vi "SET Project Editor.vi"() -> ()   [LabVIEW 2013]
uses:
  Lib/Splash/SET_Splash.lvlib
panel:
  out "Status":string=" "
  # "SET Localization Project Editor"
  # "Edit-time language switching toolkit for NI LabVIEW\"! 2013"
  # "Version 0.4.0"
  # "Copyright © 2014, Ryan Porter. All rights reserved."
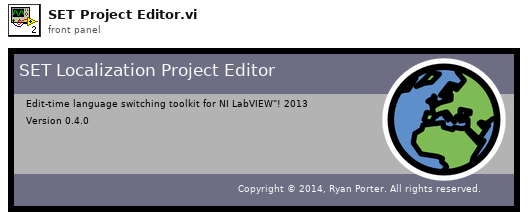
[diagram p1: front panel]
types:
  T1 = enum32{"Invalid", "Standard", "Closed", "Hidden", "Minimized", "Maximized"}
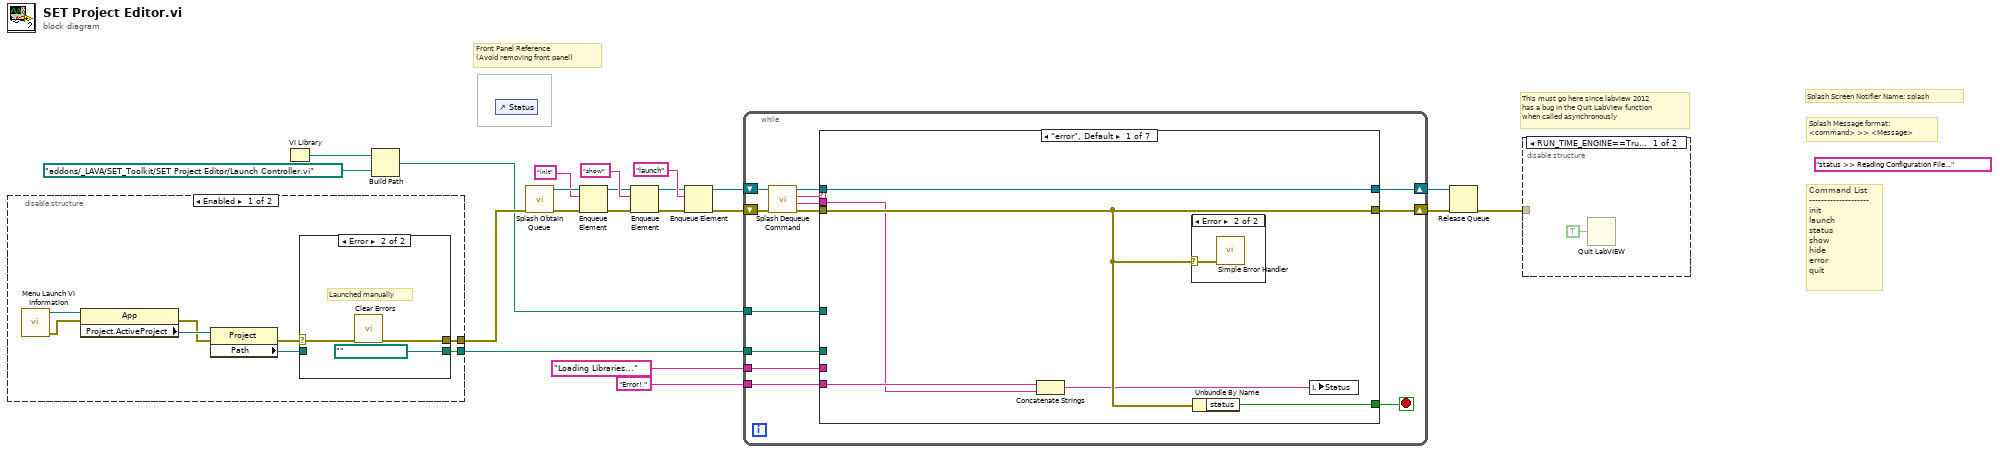
[diagram p0: block diagram]
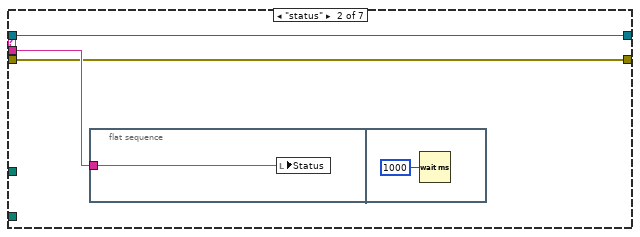
[diagram p3: hidden frame]
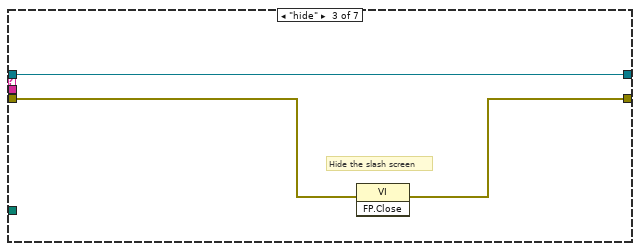
[diagram p4: hidden frame]
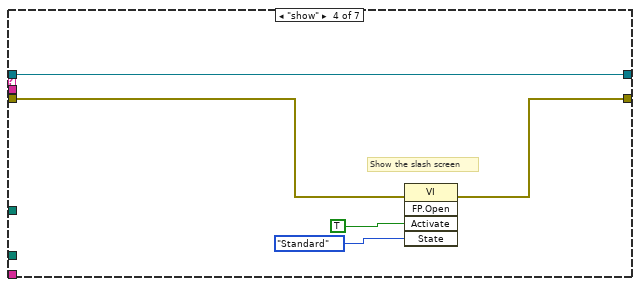
[diagram p5: hidden frame]
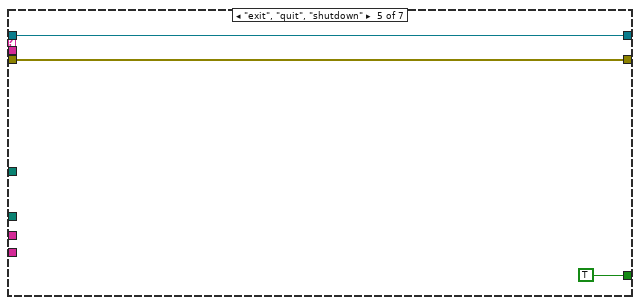
[diagram p6: hidden frame]
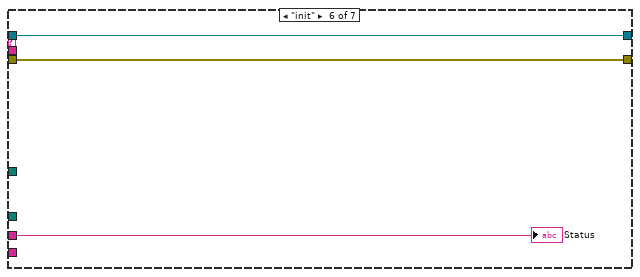
[diagram p7: hidden frame]
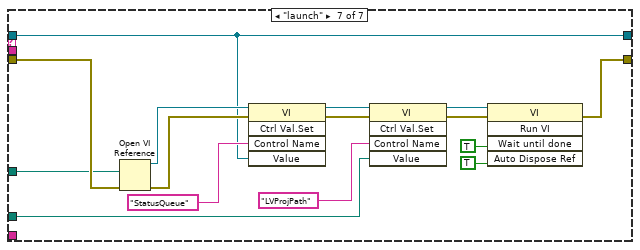
[diagram p8: hidden frame]
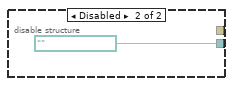
[diagram p11: hidden frame]
diagram:
  (unwired) "status >> Reading Configuration File..."
  # "Front Panel Reference\n(Avoid removing front panel)"
  # "Splash Screen Notifier Name: splash"
  # "Command List\n--------------------\ninit\nlaunch\nstatus\nshow\nhide\nerror\nquit"
  # "Splash Message format:\n<command> >> <Message>"
  # "This must go here since labview 2012\nhas a bug in the Quit LabView function\nwhen called asynchronously"
  n1 = disable-structure shown="Enabled" {
    disable-tunnel: [w29 _] -> w5
    disable-tunnel: [w28 path "" ("Path")] -> w4
    frame Enabled {
      n2 = call <vilib>:"Menu Launch VI Information.vi"() -> ("error out"=w24:errorcluster, "Menu Launch:App"=w25:refnum<vi>)  [unwired: 1 in, 9 out]
      n3 = property class="App"(reference=w25, error in=w24) -> (error out=w26:errorcluster, "Project.ActiveProject"=w27:refnum<vi>)  [unwired: 1 out]
      n4 = property class="Project"(reference=w27, error in=w26) -> (error out=w22:errorcluster, "Path"=w23:path)  [unwired: 1 out]
      n5 = case shown="Error" w22 {
        selector: w22 -> [w30 w33]
        tunnel: [w31 path "" ("Path")] -> w28
        tunnel: [w30 w32] -> w29
        tunnel: w23 -> [w31 _]
        frame No Error {
          # "Launch From Tools Menu"
        }
        frame Error {
          # "Launched manually"
          n6 = call <vilib>:"Clear Errors.vi"("error in (no error)"=w33) -> ("error out"=w32:errorcluster)  [unwired: 6 in]
        }
      }
    }
    frame Disabled {
    }
  }
  n7 = VI Library() -> (path=w3:path)
  n8 = Build Path(base path=w3, name or relative path=path "addons/_LAVA/SET_Toolkit/SET Project Editor/Launch Controller.vi" ("vi path")) -> (appended path=w1:path)
  n9 = control-ref of="Status"() -> ()  [unwired: 1 out]
  n10 = call "Splash Obtain Queue.vi"("error in (no error)"=w5) -> ("error out"=w21:errorcluster, "splash queue out"=w20:refnum<queue>)  [unwired: 9 in]
  n11 = Enqueue Element(queue=w20, element="init" ("notification"), error in (no error)=w21) -> (queue out=w11:refnum<queue>, error out=w12:errorcluster)  [unwired: 1 in, 1 out]
  n12 = Enqueue Element(queue=w11, element="show", error in (no error)=w12) -> (queue out=w15:refnum<queue>, error out=w16:errorcluster)  [unwired: 1 in, 1 out]
  n13 = Enqueue Element(queue=w15, element="launch", error in (no error)=w16) -> (queue out=w18:refnum<queue>, error out=w14:errorcluster)  [unwired: 1 in, 1 out]
  n14 = while {
    tunnel: "Loading Libraries..." ("notification") -> [w48]
    tunnel: "Error! " ("Current action") -> [w47]
    shift-right: [w46] -> w9
    shift-left: w18 -> [w45]
    shift-right: [w39] -> w19
    shift-left: w14 -> [w44]
    tunnel: w1 -> [w37]
    tunnel: w4 -> [w36]
    stop <- w38 stop-if-true
    n15 = call "Splash Dequeue Command.vi"("error in (no error)"=w44, "Splash Queue in"=w45) -> ("error out"=w41:errorcluster, "Message"=w40:string, "Command"=w42:string, "Splash Queue out"=w43:refnum<queue>)  [unwired: 6 in]
    n16 = case shown="\"error\", Default" w42 {
      tunnel: w48 -> [_ _ _ _ _ w72 _]
      tunnel: w43 -> [w54 w57 w63 w68 w69 w74 w76]
      tunnel: w41 -> [w52 w56 w62 w65 w70 w73 w79]
      tunnel: w40 -> [w50 w58 _ _ _ _ _]
      tunnel: [w52 w56 w61 w64 w70 w73 w75] -> w39
      tunnel: w47 -> [w51 _ _ _ _ _ _]
      tunnel: [w54 w57 w63 w68 w69 w74 w76] -> w46
      tunnel: [w53 _ _ _ TRUE _ _] -> w38
      tunnel: w37 -> [_ _ _ _ _ _ w78]
      tunnel: w36 -> [_ _ _ _ _ _ w77]
      frame "error", Default {
        n17 = Concatenate Strings(w51, w50) -> (w49:string)
        n18 = case shown="Error" w52 {
          selector: w52 -> [_ w55]
          frame No Error {
          }
          frame Error {
            n19 = call <vilib>:"Simple Error Handler.vi"("error in (no error)"=w55) -> ()  [unwired: 4 in, 5 out]
          }
        }
        n20 = Unbundle By Name(w52) -> ("status"=w53:bool)
        n21 = local write "Status"(w49) -> ()
      }
      frame "status" {
        n22 = flat-sequence {
          tunnel: w58 -> [w59]
          frame #0 {
            n23 = local write "Status"(w59) -> ()
          }
          frame #1 {
            n24 = Wait (ms)(milliseconds to wait=u32 1000) -> ()  [unwired: 1 out]
          }
        }
      }
      frame "hide" {
        # "Hide the slash screen"
        n25 = invoke class="VI" method="FP.Close"(error in=w62) -> (error out=w61:errorcluster)  [unwired: 2 in, 2 out]
      }
      frame "show" {
        # "Show the slash screen"
        n26 = invoke class="VI" method="FP.Open"(error in=w65, "Activate"=TRUE ("Activate?"), "State"=T1."Standard") -> (error out=w64:errorcluster)  [unwired: 2 in, 4 out]
      }
      frame "exit", "quit", "shutdown" {
      }
      frame "init" {
        "Status" <- w72
      }
      frame "launch" {
        n27 = Open VI Reference(vi path=w78, error in (no error)=w79) -> (vi reference=w87:refnum<vi>, error out=w81:errorcluster)  [unwired: 4 in]
        n28 = invoke class="VI" method="Ctrl Val.Set"(reference=w87, error in=w81, "Control Name"="StatusQueue", "Value"=w76) -> (reference out=w85:refnum<vi>, error out=w82:errorcluster)  [unwired: 1 in, 3 out]
        n29 = invoke class="VI" method="Ctrl Val.Set"(reference=w85, error in=w82, "Control Name"="LVProjPath", "Value"=w77) -> (reference out=w84:refnum<vi>, error out=w83:errorcluster)  [unwired: 1 in, 3 out]
        n30 = invoke class="VI" method="Run VI"(reference=w84, error in=w83, "Wait until done"=TRUE ("Wait Until Done"), "Auto Dispose Ref"=TRUE ("Auto Dispose Reference")) -> (error out=w75:errorcluster)  [unwired: 1 in, 4 out]
      }
    }
  }
  n31 = Release Queue(queue=w9, error in (no error)=w19) -> (error out=w8:errorcluster)  [unwired: 1 in, 2 out]
  n32 = disable-structure shown="RUN_TIME_ENGINE==True" {
    disable-tunnel: w8 -> [_ _]
    frame condition #0 {
      n33 = Quit LabVIEW(quit? (T)=TRUE) -> ()
    }
    frame condition #1 (active) {
    }
  }
